vi "RunScriptClient.vi"(1 "Immediate":bool, 2 "Filename":path) -> (0 "Error":bool)   [LabVIEW 2014]
doc: "Use this template to build a standard state machine design pattern. Each state executes code and determines which state to transition to. Contrast this design pattern with the user interface event pattern, in which code executes in response to user actions. Contrast this design pattern also with the queued message handler pattern, in which each message handling code can queue zero or more new messages."
uses:
  globals/AzCamGlobals.vi
panel:
  in  "Close":bool
  in  "Run":bool
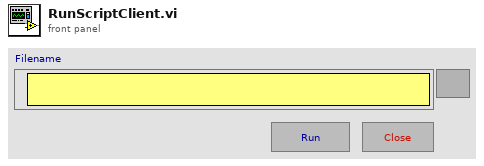
[diagram p1: front panel]
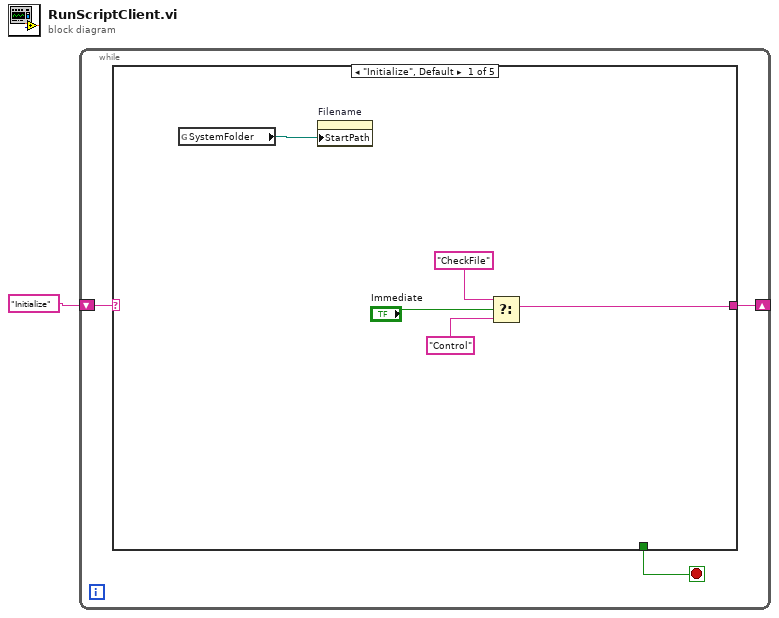
[diagram p0: block diagram]
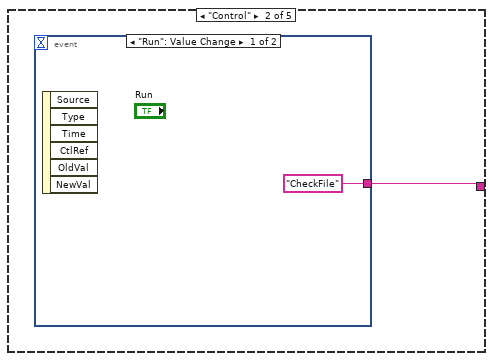
[diagram p2: hidden frame]
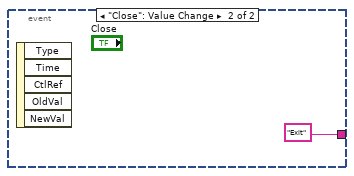
[diagram p3: hidden frame]
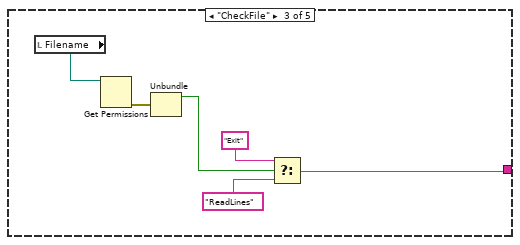
[diagram p4: hidden frame]
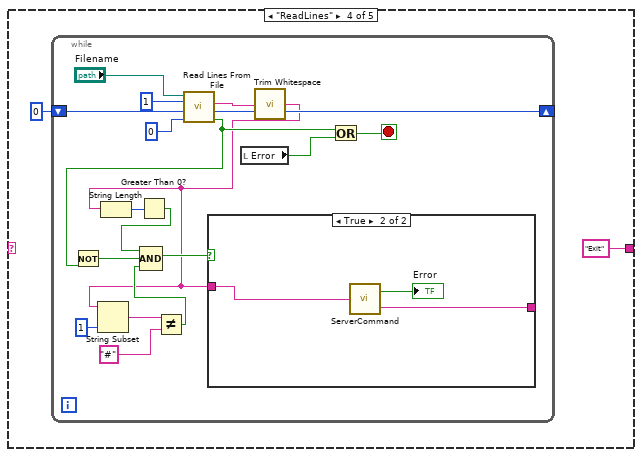
[diagram p5: hidden frame]
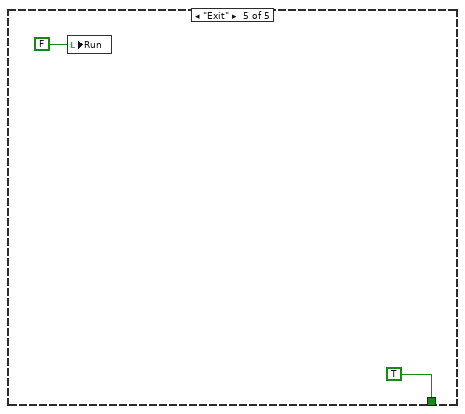
[diagram p7: hidden frame]
diagram:
  n1 = while {
    shift-right: [w2] -> _
    shift-left: "Initialize" -> [w3]
    stop <- w4 stop-if-true
    n2 = case shown="\"Initialize\", Default" w3 {
      tunnel: [_ _ _ _ TRUE] -> w4
      tunnel: [w6 w10 w13 "Exit" _] -> w2
      frame "Initialize", Default {
        n3 = global read "AzCamGlobals.vi" "SystemFolder"() -> (w5:path)
        n4 = property on="Filename" class="Path"("StartPath"=w5) -> ()  [unwired: 2 in, 2 out]
        n5 = Select(t="CheckFile", s="Immediate", f="Control") -> (s? t:f=w6:string)
      }
      frame "Control" {
        n6 = event shown="[0] \"Run\": Value Change" {
          selector: _ -> [_ _]
          dyn-events: _ -> [_ _]
          timeout: _ -> [_ _]
          tunnel: ["CheckFile" "Exit"] -> w10
          event "Run": Value Change {
            n7 = event-data() -> ()  [unwired: 1 in, 6 out]
          }
          event "Close": Value Change {
            n8 = event-data() -> ()  [unwired: 1 in, 5 out]
          }
        }
      }
      frame "CheckFile" {
        n9 = local read "Filename"() -> (w18:path)
        n10 = Get Permissions(11:w18) -> (0:w17:errorcluster)  [unwired: 1 in, 4 out]
        n11 = Unbundle(w17) -> ("status"=w16:bool)  [unwired: 2 out]
        n12 = Select(t="Exit", s=w16, f="ReadLines") -> (s? t:f=w13:string)
      }
      frame "ReadLines" {
        n13 = while {
          shift-right: [w36] -> _
          shift-left: 0 ("mark after read (chars.)") -> [w35]
          stop <- w29 stop-if-true
          n14 = call <vilib>:"Read Lines From File.vi"("file path (dialog if empty)"="Filename", "number of lines (all:-1)"=1, "start of read offset (chars.:0)"=w35, "[max characters per line]  (no limit:0)"=0) -> ("line string"=w22:string, "mark after read (chars.)"=w36:i32, "EOF?"=w28:bool)  [unwired: 2 in, 1 out]
          n15 = Not(x=w28) -> (.not. x?=w30:bool)
          n16 = local read "Error"() -> (w27:bool)
          n17 = call <vilib>:"Trim Whitespace.vi"("string"=w22) -> ("trimmed string"=w21:string)  [unwired: 1 in]
          n18 = String Subset(string=w21, length (rest)=1 ("length (rest)")) -> (substring=w25:string)  [unwired: 1 in]
          n19 = String Length(string=w21) -> (length=w33:i32)
          n20 = Greater Than 0?(x=w33) -> (x > 0?=w31:bool)
          n21 = Not Equal?(x=w25, y="#") -> (x != y?=w23:bool)
          n22 = Compound Arithmetic op=AND(w31, w30, w23) -> (w32:bool)
          n23 = case shown="True" w32 {
            tunnel: w21 -> [_ w39]
            tunnel: [_ w40] -> _
            frame False {
            }
            frame True {
              n24 = call "ServerCommand.vi"("Command"=w39) -> ("Error"=→"Error":bool, "Reply"=w40:string)
            }
          }
          n25 = Or(x=w28, y=w27) -> (x .or. y?=w29:bool)
        }
      }
      frame "Exit" {
        n26 = local write "Run"(FALSE ("Read")) -> ()
      }
    }
  }
